vi "Format RIO Device Name.vi"(8 "error in (no error)":errorcluster, 11 "FPGA CD Ref":T1 format="%.0x") -> (0 "error out":errorcluster, 3 "String":string)   [LabVIEW 2016, in "FPGA Resource Manager System Definition.lvlib"]
uses:
  FPGA Resource Manager System Definition.lvlib
  <vilib>/NI Veristand/Custom Device API/Custom Device Item Ref.ctl
  <vilib>/NI Veristand/Custom Device API/Get Item Property (String).vi
  <vilib>/NI VeriStand/Custom Device API/Custom Device API.lvlib
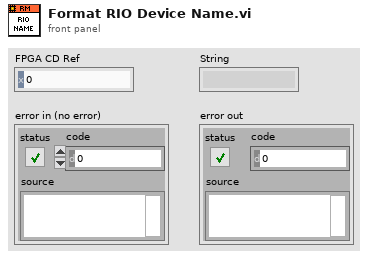
[diagram p1: front panel]
types:
  T1 = typedef "Custom Device API.lvlib/Custom Device Item Ref.ctl" = u64
  T2 = typedef "Custom Device API.lvlib/Custom Device Item Info.ctl" = cluster{"Name":string, "Is Channel":bool, "GUID":string, "Is Waveform":bool}
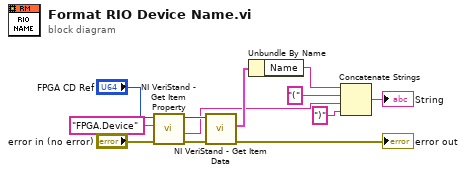
[diagram p0: block diagram]
diagram:
  n1 = call-poly <vilib>:"NI VeriStand - Get Item Property.vi"("error in (no error)"="error in (no error)", "Property Name"="FPGA.Device", "Item Ref in"="FPGA CD Ref") -> ("error out"=w10:errorcluster, "Value"=w3:string, "Item Ref out"=w6:T1)  [unwired: 5 in, 1 out]
  n2 = call <vilib>:"NI VeriStand - Get Item Data.vi"("error in (no error)"=w10, "Item Ref in"=w6) -> ("error out"=→"error out":errorcluster, "Item Info"=w7:T2)  [unwired: 6 in, 2 out]
  n3 = Unbundle By Name(w7) -> ("Name"=w8:string)
  n4 = Concatenate Strings(w8, "(" ("string"), w3, ")" ("string")) -> (→"String":string)
